vi "Skip Display Images.vi"(0 "fpga interface in":refnum<k20>, 5 "display channel number":i32, 7 "image metadata":T1[](array[typedef]), 11 "error in (no error)":errorcluster) -> (4 "fpga interface out":refnum<k20>, 15 "error out":errorcluster)   [LabVIEW 2023, in "GettingStarted_Common_148X_Host.lvlib"]
uses:
  GettingStarted_Common_148X_Host.lvlib
  FPGA/Common/Types/Image Metadata.ctl
  <instrlib>/FlexRIO/CSI-2/v2/Common/Types/LLP Data Type.ctl
  FPGA/Common/GettingStarted_Common_148X_FPGA.lvlib
  <instrlib>/FlexRIO/CSI-2/v2/Common/NI CSI-2 API Common v2.lvlib
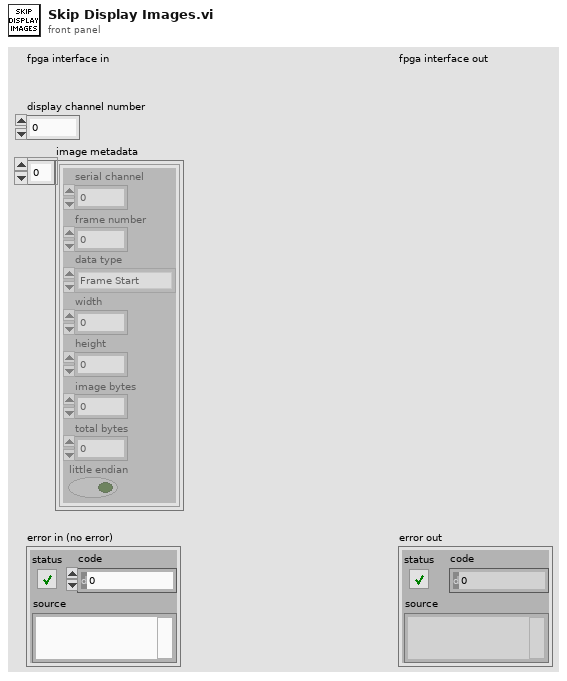
[diagram p1: front panel]
types:
  T1 = typedef "GettingStarted_Common_148X_FPGA.lvlib/Image Metadata.ctl" = cluster{"serial channel":fxp<+,3,3>, "frame number":u16, "data type":T2, "width":u16, "height":u16, "image bytes":u32, "total bytes":u32, "little endian":bool}
  T2 = typedef "NI CSI-2 API Common v2.lvlib/LLP Data Type.ctl" = enum8{"Frame Start", "Frame End", "Line Start", "Line End", "End of Transmission", "Reserved 0", "Reserved 1", "Reserved 2", "Generic Short Packet 1", "Generic Short Packet 2", "Generic Short Packet 3", "Generic Short Packet 4", "Generic Short Packet 5", "Generic Short Packet 6", "Generic Short Packet 7", "Generic Short Packet 8", "Null", "Blanking Data", "Embedded 8-bit non Image Data", "Generic Long Packet 1", "Generic Long Packet 2", "Generic Long Packet 3", "Generic Long Packet 4", "Reserved 3", "YUV420 8-bit", "YUV420 10-bit", "Legacy YUV420 8-bit", "Reserved 4", "YUV420 8-bit Chroma Shifted", "YUV420 10-bit Chroma Shifted", "YUV422 8-bit", "YUV422 10-bit", "RGB444", "RGB555", "RGB565", "RGB666", "RGB888", "Reserved 5", "Reserved 6", "RAW 24", "RAW 6", "RAW 7", "RAW 8", "RAW 10", "RAW 12", "RAW 14", "RAW 16", "RAW 20", "User Defined 8-bit Data 1", "User Defined 8-bit Data 2", "User Defined 8-bit Data 3", "User Defined 8-bit Data 4", "User Defined 8-bit Data 5", "User Defined 8-bit Data 6", "User Defined 8-bit Data 7", "User Defined 8-bit Data 8", "USL Command", "Reserved 7", "Reserved 8", "Reserved 9", "Reserved 10", "Reserved 11", "Reserved 12", "LRTE EPD Spacer"}
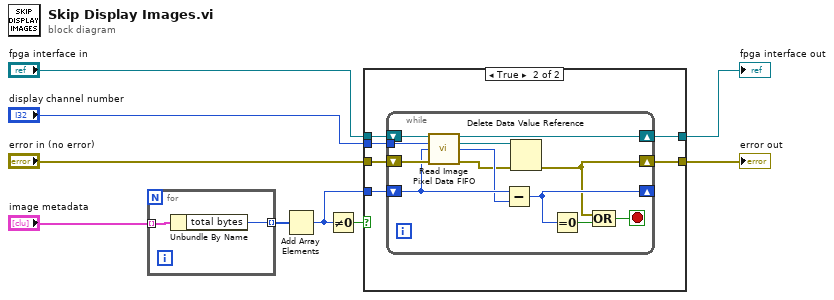
[diagram p0: block diagram]
diagram:
  n1 = for {
    tunnel: "image metadata" -> [w11] mode=indexing
    tunnel: [w10] -> w5 mode=indexing
    n2 = Unbundle By Name(w11) -> ("total bytes"=w10:u32)
  }
  n3 = Add Array Elements(numeric array=w5) -> (sum=w1:u32)
  n4 = Not Equal To 0?(x=w1) -> (x != 0?=w2:bool)
  n5 = case shown="True" w2 {
    tunnel: "error in (no error)" -> [w13 w19]
    tunnel: [w13 w18] -> w8
    tunnel: [w12 w17] -> w7
    tunnel: "fpga interface in" -> [w12 w16]
    tunnel: w1 -> [_ w15]
    tunnel: "display channel number" -> [_ w14]
    frame False {
    }
    frame True {
      n6 = while {
        tunnel: w14 -> [w29]
        shift-right: [w30] -> w17
        shift-left: w16 -> [w31]
        shift-right: [w22] -> w18
        shift-left: w19 -> [w28]
        shift-right: [w25] -> _
        shift-left: w15 -> [w27]
        stop <- w23 stop-if-true
        n7 = call "Read Image Pixel Data FIFO.vi"("fpga inteface in"=w31, "display channel number"=w29, "number of elements"=w27, "error in (no error)"=w28) -> ("fpga interface out"=w30:refnum<k20>, "image pixel data region"=w21:refnum<data-value>, "elements in region"=w26:u32, "error out"=w20:errorcluster)  [unwired: 7 in, 1 out]
        n8 = Subtract(x=w27, y=w26) -> (x-y=w25:u32)
        n9 = Delete Data Value Reference(data value reference=w21, error in=w20) -> (error out=w22:errorcluster)  [unwired: 1 out]
        n10 = Equal To 0?(x=w25) -> (x = 0?=w24:bool)
        n11 = Compound Arithmetic op=OR(w22, w24) -> (w23:bool)
      }
    }
  }
  "error out" <- w8
  "fpga interface out" <- w7
